vi "DriveForwardDistance.vi"(7 "Timeout":dbl, 8 "Error In":errorcluster, 9 "Initation?":bool, 10 "MaxSpeed":dbl, 11 "Distance":dbl) -> (0 "Error Out":errorcluster, 2 "Succesful":bool, 3 "Finished":bool)   [LabVIEW 2020]
uses:
  <vilib>/Utility/semaphor.llb/Obtain Semaphore Reference.vi
  <vilib>/Rock Robotics/WPI/ThirdParty/JAS_Junk/TrajLib/Timer_Reset.vi
  DriveGlobals.vi
  <vilib>/Rock Robotics/WPI/ThirdParty/JAS_Junk/TrajLib/Trajectory_Library.lvlib
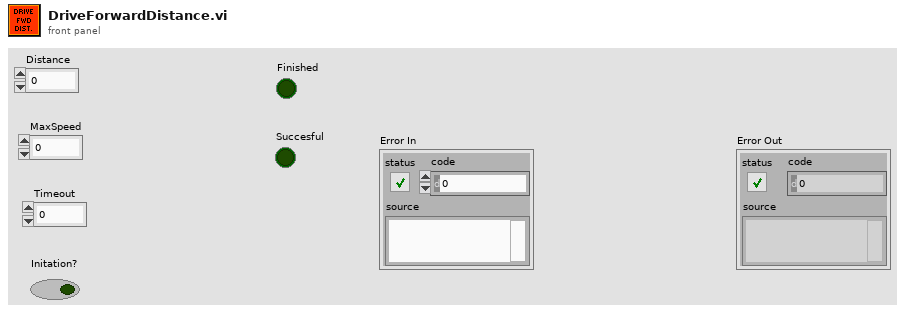
[diagram p1: front panel]
types:
  T1 = typedef "Trajectory_Library.lvlib/TIMER.ctl" = cluster{"StartTime":dbl, "Accumulated TIme":dbl, "Running":bool, "semaphore":T2}
  T2 = typedef "Semaphore RefNum" = refnum<k1>
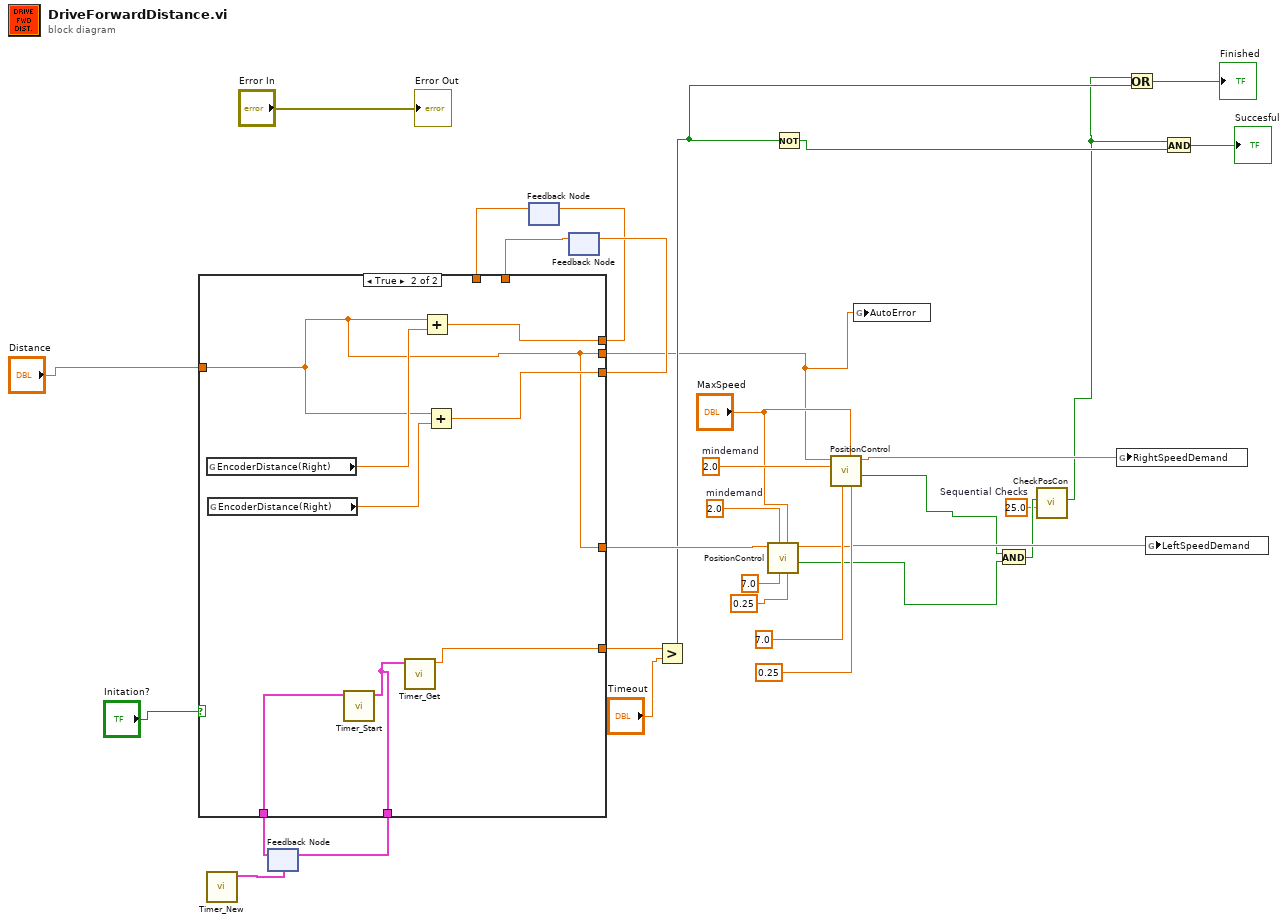
[diagram p0: block diagram]
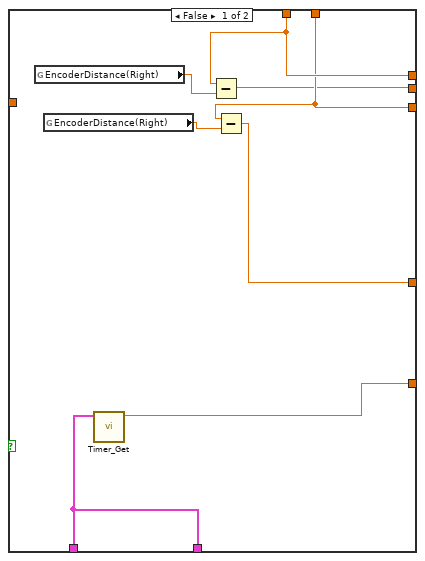
[diagram p2: hidden frame]
diagram:
  w1 = 25.0  # Sequential Checks
  w17 = 2.0  # mindemand
  w13 = 2.0  # mindemand
  n1 = call <vilib>:"Timer_New.vi"() -> ("TIMER"=w10:T1)  [unwired: 11 in]
  n2 = feedback #1(w10) -> (w30:T1)
  n3 = feedback #2() -> (w24:dbl)  [unwired: 1 in]
  n4 = feedback #3() -> (w26:dbl)  [unwired: 1 in]
  n5 = case shown="True" "Initation?" {
    tunnel: w30 -> [w33 w42]
    tunnel: "Distance" -> [_ w43]
    tunnel: w24 -> [w40 _]
    tunnel: [w40 w46] -> w25
    tunnel: w26 -> [w38 _]
    tunnel: [w38 w45] -> w27
    tunnel: [w36 w44] -> w20
    tunnel: [w35 w43] -> w16
    tunnel: [w34 w43] -> w4
    tunnel: [w33 w41] -> w9
    frame False {
      n6 = global read "DriveGlobals.vi" "EncoderDistance(Right)"() -> (w39:dbl)
      n7 = global read "DriveGlobals.vi" "EncoderDistance(Right)"() -> (w37:dbl)
      n8 = call <vilib>:"Timer_Get.vi"("TIMER"=w33) -> ("CurrentTImer"=w36:dbl)  [unwired: 10 in]
      n9 = Subtract(x=w40, y=w39) -> (x-y=w34:dbl)
      n10 = Subtract(x=w38, y=w37) -> (x-y=w35:dbl)
    }
    frame True {
      n11 = global read "DriveGlobals.vi" "EncoderDistance(Right)"() -> (w47:dbl)
      n12 = global read "DriveGlobals.vi" "EncoderDistance(Right)"() -> (w48:dbl)
      n13 = call <vilib>:"Timer_Start.vi"("in Timer"=w42) -> ("out Timer"=w41:T1)  [unwired: 10 in]
      n14 = call <vilib>:"Timer_Get.vi"("TIMER"=w41) -> ("CurrentTImer"=w44:dbl)  [unwired: 10 in]
      n15 = Add(x=w43, y=w47) -> (x+y=w46:dbl)
      n16 = Add(x=w43, y=w48) -> (x+y=w45:dbl)
    }
  }
  n17 = feedback-in #1(w9) -> ()
  n18 = feedback-in #2(w25) -> ()
  n19 = feedback-in #3(w27) -> ()
  n20 = Greater?(x=w20, y="Timeout") -> (0:w7:bool)
  n21 = call "PositionControl.vi"("deadband"=0.25, "maxdemand"="MaxSpeed", "threshold"=7.0, "mindemand"=w17, "Error"=w16) -> ("on target"=w6:bool, "output variable"=w12:dbl)  [unwired: 5 in]
  n22 = Not(x=w7) -> (.not. x?=w22:bool)
  n23 = call "PositionControl.vi"("deadband"=0.25, "maxdemand"="MaxSpeed", "threshold"=7.0, "mindemand"=w13, "Error"=w4) -> ("on target"=w5:bool, "output variable"=w11:dbl)  [unwired: 5 in]
  n24 = global write "DriveGlobals.vi" "AutoError"(w4) -> ()
  n25 = And(x=w5, y=w6) -> (x .and. y?=w3:bool)
  n26 = call "CheckPosCon.vi"("Sequential Checks"=w1, "WasRight"=w3) -> ("We made It"=w2:bool)  [unwired: 9 in]
  n27 = global write "DriveGlobals.vi" "RightSpeedDemand"(w11) -> ()
  n28 = Or(x=w2, y=w7) -> (x .or. y?=→"Finished":bool)
  n29 = global write "DriveGlobals.vi" "LeftSpeedDemand"(w12) -> ()
  n30 = And(x=w2, y=w22) -> (x .and. y?=→"Succesful":bool)
  "Error Out" <- "Error In"
